vi "LN2 Saturation Lookup.vi"(9 "error in":errorcluster, 11 "Temperature":dbl=-280.0) -> (1 "error out":errorcluster, 2 "Saturation Density":dbl, 3 "Saturation Pressure":dbl)   [LabVIEW 2024]
uses:
  <vilib>/Utility/file.llb/Read Delimited Spreadsheet (DBL).vi
panel:
  in  "Lookup Table":dbl[][](array[numeric])=[[-340.0, 3.2401, 53.277, 0.01877], [-339.0, 3.5466, 53.131, 0.018821], [-338.0, 3.8757, 52.985, 0.018873], [-337.0, 4.2285, 52.839, 0.018925], [-336.0, 4.6063, 52.692, 0.018978], [-335.0, 5.0104, 52.544, 0.019032], [-334.0, 5.4418, 52.396, 0.019085], [-333.0, 5.902, 52.247, 0.01914], [-332.0, 6.3921, 52.098, 0.019195], [-331.0, 6.9136, 51.948, 0.01925], [-330.0, 7.4677, 51.797, 0.019306], [-329.0, 8.0558, 51.646, 0.019363], [-328.0, 8.6793, 51.494, 0.01942], [-327.0, 9.3396, 51.341, 0.019478], [-326.0, 10.038, 51.188, 0.019536], [-325.0, 10.776, 51.034, 0.019595], [-324.0, 11.556, 50.88, 0.019654], [-323.0, 12.378, 50.724, 0.019714], [-322.0, 13.244, 50.568, 0.019775], [-321.0, 14.156, 50.412, 0.019837], [-320.0, 15.115, 50.254, 0.019899], [-319.0, 16.123, 50.096, 0.019962], [-318.0, 17.181, 49.937, 0.020025], [-317.0, 18.292, 49.778, 0.020089], [-316.0, 19.455, 49.617, 0.020154], [-315.0, 20.674, 49.456, 0.02022], [-314.0, 21.95, 49.294, 0.020287], [-313.0, 23.284, 49.131, 0.020354], [-312.0, 24.679, 48.967, 0.020422], [-311.0, 26.135, 48.802, 0.020491], [-310.0, 27.654, 48.636, 0.020561], [-309.0, 29.239, 48.47, 0.020631], [-308.0, 30.891, 48.302, 0.020703], [-307.0, 32.611, 48.134, 0.020775], [-306.0, 34.401, 47.964, 0.020849], [-305.0, 36.264, 47.794, 0.020923], [-304.0, 38.2, 47.622, 0.020999], [-303.0, 40.212, 47.45, 0.021075], [-302.0, 42.3, 47.276, 0.021152], [-301.0, 44.468, 47.101, 0.021231], [-300.0, 46.717, 46.925, 0.021311], [-299.0, 49.048, 46.748, 0.021391], [-298.0, 51.464, 46.569, 0.021473], [-297.0, 53.966, 46.39, 0.021556], [-296.0, 56.556, 46.209, 0.021641], [-295.0, 59.235, 46.027, 0.021727], [-294.0, 62.006, 45.843, 0.021814], [-293.0, 64.871, 45.658, 0.021902], [-292.0, 67.83, 45.472, 0.021992], [-291.0, 70.887, 45.284, 0.022083], [-290.0, 74.043, 45.094, 0.022176], [-289.0, 77.299, 44.903, 0.02227], [-288.0, 80.658, 44.71, 0.022366], [-287.0, 84.122, 44.516, 0.022464], [-286.0, 87.692, 44.32, 0.022563], [-285.0, 91.37, 44.122, 0.022664], [-284.0, 95.158, 43.922, 0.022767], [-283.0, 99.059, 43.721, 0.022872], [-282.0, 103.07, 43.517, 0.022979], [-281.0, 107.2, 43.312, 0.023088], [-280.0, 111.45, 43.104, 0.0232], [-279.0, 115.82, 42.894, 0.023313], [-278.0, 120.31, 42.682, 0.023429], [-277.0, 124.92, 42.467, 0.023548], [-276.0, 129.66, 42.25, 0.023669], [-275.0, 134.53, 42.03, 0.023792], [-274.0, 139.52, 41.808, 0.023919], [-273.0, 144.65, 41.583, 0.024048], [-272.0, 149.91, 41.355, 0.024181], [-271.0, 155.31, 41.124, 0.024317], [-270.0, 160.84, 40.89, 0.024456], [-269.0, 166.52, 40.653, 0.024599], [-268.0, 172.34, 40.412, 0.024745], [-267.0, 178.3, 40.168, 0.024896], [-266.0, 184.41, 39.919, 0.02505], [-265.0, 190.66, 39.667, 0.02521], [-264.0, 197.07, 39.411, 0.025374], [-263.0, 203.63, 39.15, 0.025543], [-262.0, 210.35, 38.885, 0.025717], [-261.0, 217.22, 38.614, 0.025897], [-260.0, 224.25, 38.339, 0.026083], [-259.0, 231.45, 38.058, 0.026276], [-258.0, 238.81, 37.771, 0.026475], [-257.0, 246.34, 37.478, 0.026682], [-256.0, 254.04, 37.179, 0.026897], [-255.0, 261.91, 36.872, 0.027121], [-254.0, 269.96, 36.558, 0.027354], [-253.0, 278.19, 36.236, 0.027597], [-252.0, 286.6, 35.904, 0.027852], [-251.0, 295.19, 35.564, 0.028118], [-250.0, 303.97, 35.213, 0.028399], [-249.0, 312.94, 34.851, 0.028694], [-248.0, 322.11, 34.476, 0.029006], [-247.0, 331.47, 34.087, 0.029336], [-246.0, 341.04, 33.683, 0.029688], [-245.0, 350.81, 33.263, 0.030064], [-244.0, 360.79, 32.822, 0.030467], [-243.0, 370.98, 32.36, 0.030903], [-242.0, 381.4, 31.871, 0.031376], [-241.0, 392.04, 31.352, 0.031895], [-240.0, 402.92, 30.797, 0.03247]]
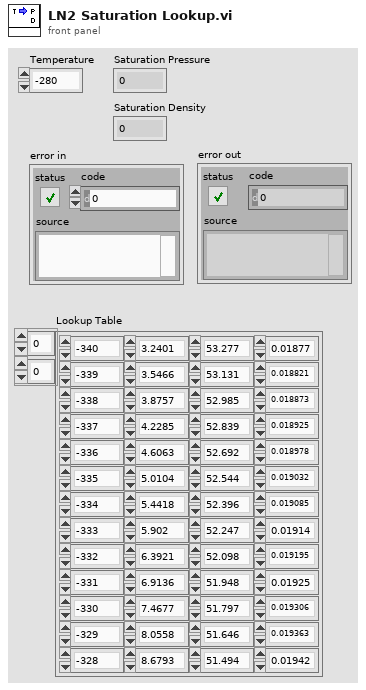
[diagram p1: front panel]
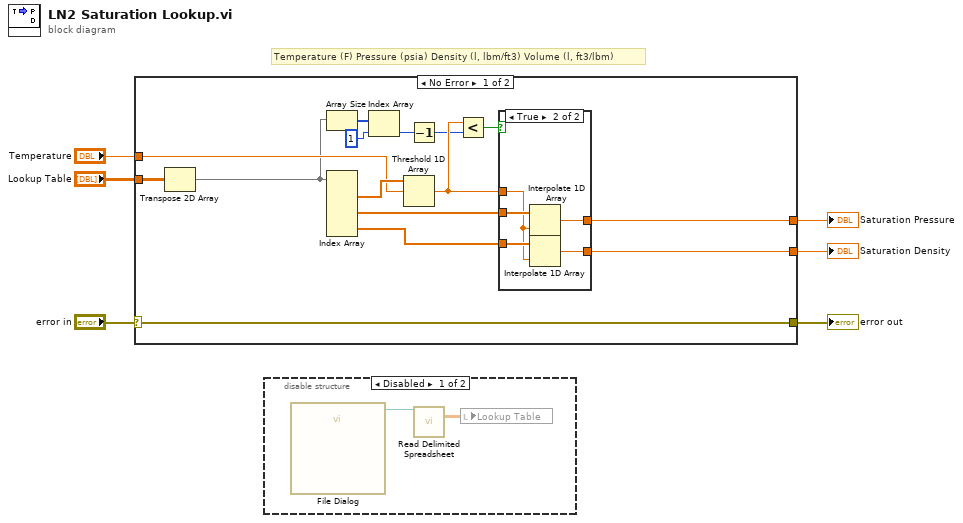
[diagram p0: block diagram]
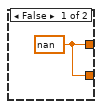
[diagram p3: hidden frame]
diagram:
  # "Temperature (F)\tPressure (psia)\tDensity (l, lbm/ft3)\tVolume (l, ft3/lbm)"
  n1 = case shown="No Error" "error in" {
    selector: "error in" -> [w21 w28]
    tunnel: [w21 w28] -> w5
    tunnel: "Temperature" -> [w17 _]
    tunnel: [w16 _] -> w3
    tunnel: "Lookup Table" -> [w20 _]
    tunnel: [w7 _] -> w1
    frame No Error {
      n2 = Transpose 2D Array(2D array=w20) -> (transposed array=w15:dbl[][])
      n3 = Array Size(array=w15) -> (size(s)=w14:i32[])
      n4 = Index Array(array=w15) -> (element #1=w19:dbl[], element #2=w18:dbl[], element #3=w8:dbl[])  [unwired: 6 in]
      n5 = Index Array(array=w14, index=1) -> (element=w13:i32)
      n6 = Threshold 1D Array(2:w17, 3:w19) -> (0:w12:dbl)  [unwired: 1 in]
      n7 = Decrement(x=w13) -> (x-1=w9:i32)
      n8 = Less?(x=w12, y=w9) -> (x < y?=w11:bool)
      n9 = case shown="True" w11 {
        tunnel: w18 -> [_ w27]
        tunnel: [w22 w26] -> w16
        tunnel: w12 -> [_ w24]
        tunnel: w8 -> [_ w25]
        tunnel: [w22 w23] -> w7
        frame False {
          w22 = nan
        }
        frame True {
          n10 = Interpolate 1D Array(1:w24, 2:w27) -> (0:w26:dbl)
          n11 = Interpolate 1D Array(1:w24, 2:w25) -> (0:w23:dbl)
        }
      }
    }
    frame Error {
    }
  }
  "Saturation Pressure" <- w3
  "error out" <- w5
  "Saturation Density" <- w1
  n12 = disable-structure shown="Disabled" {
    frame Disabled {
      n13 = call "File Dialog"() -> ("selected path"=w29:path)  [unwired: 12 in, 3 out]
      n14 = call-poly <vilib>:"Read Delimited Spreadsheet.vi"("file path (dialog if empty)"=w29) -> ("all rows"=w30:dbl[][])  [unwired: 9 in, 5 out]
      n15 = local write "Lookup Table"(w30) -> ()
    }
    frame Enabled {
    }
  }
